vi "ReadWriteN.vi"(1 "Axis":u32, 2 "Delay (ms)":i32=10, 3 "Position Input um":dbl min=0.0 max=200.0 step=0.001 format="%.4f") -> (0 "Position Read um":dbl(graph)=0.20766479492187498)   [LabVIEW 2012]
uses:
  Madlib.dll
panel:
  in  "Handle":i32
  # "This example reads the position of the nanopositioner,\ncommands it to move, and then waits for a period of \ntime for the nanopositioner to arrive at the new position.\nThis VI can be used as a SubVI for a scanning program."
  # "X = 1\nY = 2\nZ = 3"
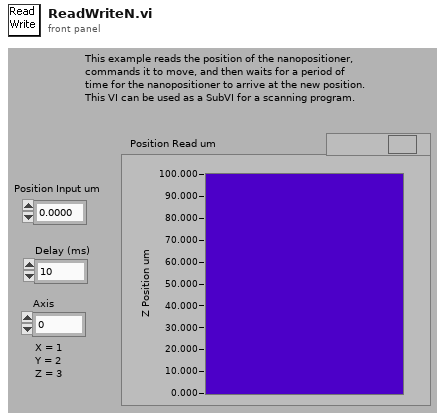
[diagram p1: front panel]
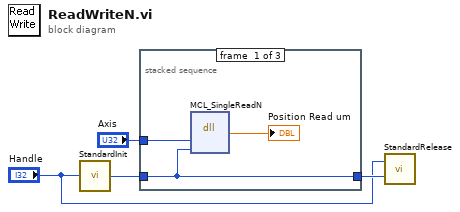
[diagram p0: block diagram]
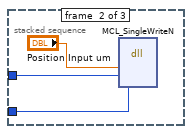
[diagram p2: hidden frame]
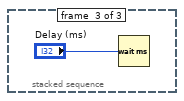
[diagram p3: hidden frame]
diagram:
  n1 = call "StandardInit.vi"("Incoming Handle"="Handle") -> ("Outgoing Handle"=w3:i32)
  n2 = stacked-sequence {
    tunnel: "Axis" -> [w7 w9 _]
    tunnel: w3 -> [w5 w8 _]
    tunnel: [w5 _ _] -> w2
    frame #0 {
      n3 = dll-call lib="C:/Users/Labview/Desktop/SRR/Madlib_x64/Labview Examples/32-bit LabView on 64-bit Windows/MADLib.dll" fn="MCL_SingleReadN"("axis"=w7, "handle"=w5) -> ("return type"=→"Position Read um":dbl)  [unwired: 5 in, 2 out]
    }
    frame #1 {
      n4 = dll-call lib="C:/Users/Labview/Desktop/SRR/Madlib_x64/Labview Examples/32-bit LabView on 64-bit Windows/MADLib.dll" fn="MCL_SingleWriteN"("position"="Position Input um", "axis"=w9, "handle"=w8) -> ()  [unwired: 7 in, 2 out]
    }
    frame #2 {
      n5 = Wait (ms)(milliseconds to wait="Delay (ms)") -> ()  [unwired: 1 out]
    }
  }
  n6 = call "StandardRelease.vi"("Outgoing Handle"=w2, "Incoming Handle"="Handle") -> ()  [unwired: 1 in]
